vi "Write Enable.vi"(8 "error in (no error)":errorcluster, 10 "Enable":refnum<k21>, 11 "DAQ HVPS in":refnum<class "DAQ HVPS.lvclass">) -> (0 "error out":errorcluster, 3 "DAQ HVPS out":refnum<class "DAQ HVPS.lvclass">)   [LabVIEW 2013, in "DAQ HVPS.lvclass"]
uses:
  DAQ HVPS.lvclass
  DAQ HVPS.lvclass/DAQ HVPS.ctl
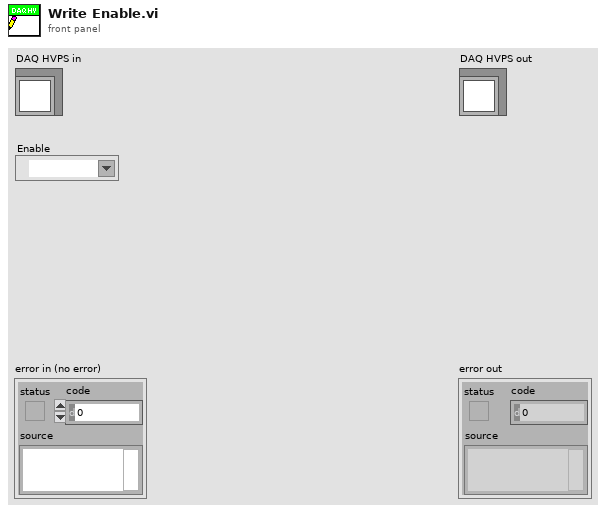
[diagram p1: front panel]
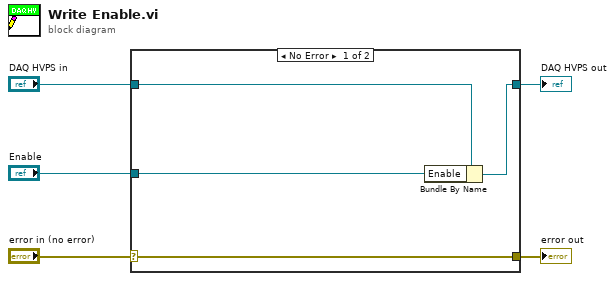
[diagram p0: block diagram]
diagram:
  n1 = case shown="No Error" "error in (no error)" {
    selector: "error in (no error)" -> [w9 w10]
    tunnel: [w9 w10] -> w4
    tunnel: [w7 w11] -> w2
    tunnel: "DAQ HVPS in" -> [w8 w11]
    tunnel: "Enable" -> [w6 _]
    frame No Error {
      n2 = Bundle By Name(cluster=w8, "Enable"=w6) -> (w7:refnum<class "DAQ HVPS.lvclass">)
    }
    frame Error {
    }
  }
  "error out" <- w4
  "DAQ HVPS out" <- w2
